vi "PlotBoatInitialize.vi"(11 "Map":enum16{"Grid"}(ring)) -> (1 "Bottom Right Pixel UTM":T1 {"North" format="%#_10f"; "East" format="%#_8f"}, 2 "Top Left Pixel UTM":T1 {"North" format="%#_10f"; "East" format="%#_8f"}, 3 "Map Image Out":T2)   [LabVIEW 2013]
doc: "This vi initializes the map image for the simulator map view\n\nMaci Crowell\n4/5/2014"
uses:
  <vilib>/vision/Image Controls.llb/IMAQ Image.ctl
  cRIO_Code/Data/TypeDefs/UTM Location.ctl
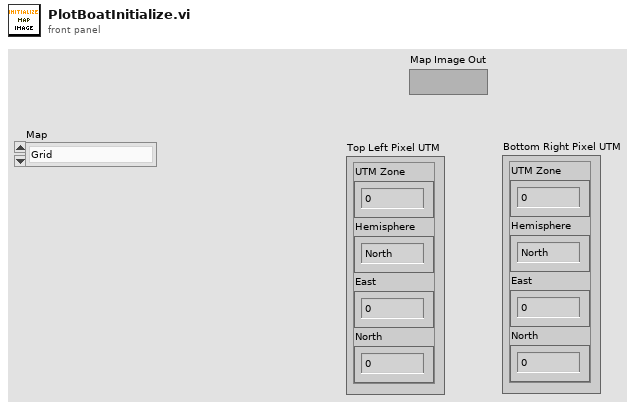
[diagram p1: front panel]
types:
  T1 = typedef "UTM Location.ctl" = cluster{"UTM Zone":dbl, "Hemisphere":enum16{"North", "South"}, "East":dbl, "North":dbl}
  T2 = typedef "IMAQ Image.ctl" = refnum<image>
  T3 = typedef "Image Type" = u32
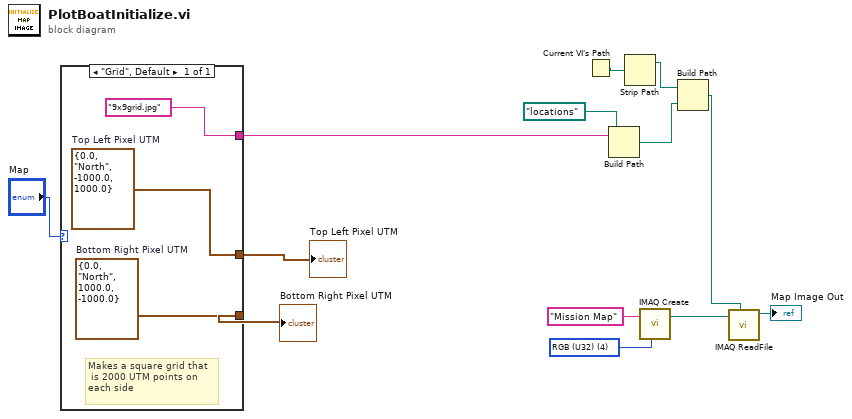
[diagram p0: block diagram]
diagram:
  w12 = T3 4 items=["Grayscale (U8)", "Grayscale (I16)", "Grayscale (SGL)", "Complex (CSG)", "RGB (U32)", "HSL (U32)", "RGB (U64)", "Grayscale (U16)"] ("Image Type")
  n1 = case shown="\"Grid\", Default" "Map" {
    tunnel: ["9x9grid.jpg"] -> w3
    tunnel: [w15] -> w2
    tunnel: [w14] -> w1
    frame "Grid", Default {
      w14 = T1 {"UTM Zone"=0.0, "Hemisphere"=enum."North", "East"=1000.0, "North"=-1000.0}  # Bottom Right Pixel UTM
      w15 = T1 {"UTM Zone"=0.0, "Hemisphere"=enum."North", "East"=-1000.0, "North"=1000.0}  # Top Left Pixel UTM
      # "Makes a square grid that\n is 2000 UTM points on \neach side"
    }
  }
  "Top Left Pixel UTM" <- w2
  "Bottom Right Pixel UTM" <- w1
  n2 = Current VI's Path() -> (path=w9:path)
  n3 = Build Path(base path=path "locations", name or relative path=w3) -> (appended path=w6:path)
  n4 = Strip Path(path=w9) -> (stripped path=w8:path)  [unwired: 1 out]
  n5 = call "IMAQ Create"("Image Name"="Mission Map", "Image Type"=w12) -> ("New Image"=w11:T2)  [unwired: 2 in, 2 out]
  n6 = Build Path(base path=w8, name or relative path=w6) -> (appended path=w5:path)
  n7 = call "IMAQ ReadFile"("File Path"=w5, "Image"=w11) -> ("Image Out"=→"Map Image Out":T2)  [unwired: 3 in, 6 out]
